vi "Module Loop.vi"(8 "error in (no error)":errorcluster, 11 "Log Manager Module in":refnum<class "Log Manager Module.lvclass">) -> (0 "error out":errorcluster, 3 "Log Manager Module out":refnum<class "Log Manager Module.lvclass">)   [LabVIEW 2023, in "VolatusData.lvlib" / "Log Manager Module.lvclass"]
uses:
  Log Manager Module.lvclass
  Volatus/Module/Module.lvclass
  Log Preparer Module/Log Preparer Module.lvclass
  Log Manager Module.lvclass/Log Manager Module.ctl
  lv-cdm/CDM-Config/ISO8601 Config.ctl
  lv-cdm/CDM-Config/Format.ctl
  lv-cdm/CDM-Config/Precision.ctl
  lv-cdm/CDM-Config/Timezone.ctl
  messages/StartLog/Data.ctl
  lv-vecto/Vecto/proto/TcpPayload/Data.ctl
  Volatus/Module/Module.lvclass/Module.ctl
  Volatus/MessageQ/MessageQ.lvclass/MessageQ.ctl
  Volatus/StringValue/StringValue.lvclass/StringValue.ctl
  Register Logger.ctl
  Volatus/MessageQ/MessageQ.lvclass
  messages/StartLog/Class/Msg.lvclass
  messages/StartLog/Class/Msg.lvclass/Msg.ctl
  Logger Ready.ctl
  messages/StopLog/Class/Msg.lvclass
  messages/StopLog/Class/Msg.lvclass/Msg.ctl
  messages/StopLog/Data.ctl
  Logger Started.ctl
  Logger Stopped.ctl
  Unregister Logger.ctl
  Volatus/Module/Self Q.vi
  Volatus/MessageQ/Send.vi
  lv-cdm/CDM-Config/ISO-8601 Format Strings.vi
  lv-promises/Promises/Promise/Promise.lvclass
  Volatus/StringValue/StringValue.lvclass
  VolatusData.lvlib
  lv-cdm/CDM-Config/CDM-Config.lvlib
  messages/StartLog/StartLog.lvlib
  lv-vecto/Vecto/proto/TcpPayload/TcpPayload.lvlib
  Log Status Value/Log Status Value.lvclass
  messages/StopLog/StopLog.lvlib
  C:/dev/volatus/mts-volatus-super/libs/lv-volatus/Volatus/Module/Module.lvclass
  C:/dev/volatus/mts-volatus-super/libs/lv-volatus/VolatusData/Log Manager Module/Log Manager Module.lvclass
  C:/dev/volatus/mts-volatus-super/libs/lv-volatus/messages/StartLog/Class/Msg.lvclass
  C:/dev/volatus/mts-volatus-super/libs/lv-protoc/LV-Proto/Message/Message.lvclass
  C:/dev/volatus/mts-volatus-super/libs/lv-volatus/messages/StopLog/Class/Msg.lvclass
panel:
  in  "Log Series":string
  in  "Log":bool
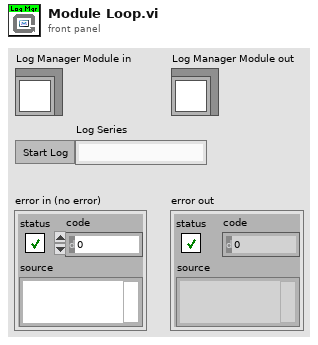
[diagram p1: front panel]
types:
  T1 = enum32{"Invalid", "Standard", "Closed", "Hidden", "Minimized", "Maximized"}
  T2 = typedef "TcpPayload.lvlib/Data.ctl" = cluster{"target_node":u32, "source_id":u32, "sequence":u32, "timestamp":i64, "type":string, "task_id":string, "payload":u8[]}
  T3 = typedef "StartLog.lvlib/Data.ctl" = cluster{"series":string, "timestamp":string, "started_by":string, "groups":string[]}
  T4 = typedef "CDM-Config.lvlib/ISO8601 Config.ctl" = cluster{"Format":T5, "Precision":T6, "Timezone":T7}
  T5 = typedef "CDM-Config.lvlib/Format.ctl" = enum16{"Extended", "Basic"}
  T6 = typedef "CDM-Config.lvlib/Precision.ctl" = enum16{"Millisecond", "Second", "Minute", "Hour", "Day"}
  T7 = typedef "CDM-Config.lvlib/Timezone.ctl" = enum16{"UTC", "Local"}
  T8 = typedef "VolatusData.lvlib/Register Logger.ctl" = cluster{"MsgQ":refnum<class "MessageQ.lvclass">, "ID":string, "Group":string}
  T9 = typedef "VolatusData.lvlib/Logger Ready.ctl" = cluster{"ID":string}
  T10 = typedef "StopLog.lvlib/Data.ctl" = cluster{"reason":string, "groups":string[]}
  T11 = typedef "VolatusData.lvlib/Logger Started.ctl" = cluster{"ID":string}
  T12 = typedef "VolatusData.lvlib/Logger Stopped.ctl" = cluster{"ID":string}
  T13 = typedef "VolatusData.lvlib/Unregister Logger.ctl" = cluster{"ID":string}
  T14 = typedef "VolatusData.lvlib/Log Manager Module.lvclass/Prep Info.ctl" = cluster{"State":T15, "Error":errorcluster}
  T15 = typedef "VolatusData.lvlib/Prep State.ctl" = enum16{"Unknown", "In Progress", "Success", "Failed"}
  T16 = typedef "VolatusData.lvlib/Log Status.ctl" = cluster{"State":T17, "Log":string, "Groups":T18[]}
  T17 = typedef "VolatusData.lvlib/Logging State.ctl" = enum16{"Idle", "Starting", "Logging", "Stopping"}
  T18 = typedef "VolatusData.lvlib/Group State.ctl" = cluster{"Group":string, "State":T19}
  T19 = typedef "VolatusData.lvlib/Logger State.ctl" = enum16{"Unknown", "Idle", "Preparing", "Ready", "Logging", "Stopping"}
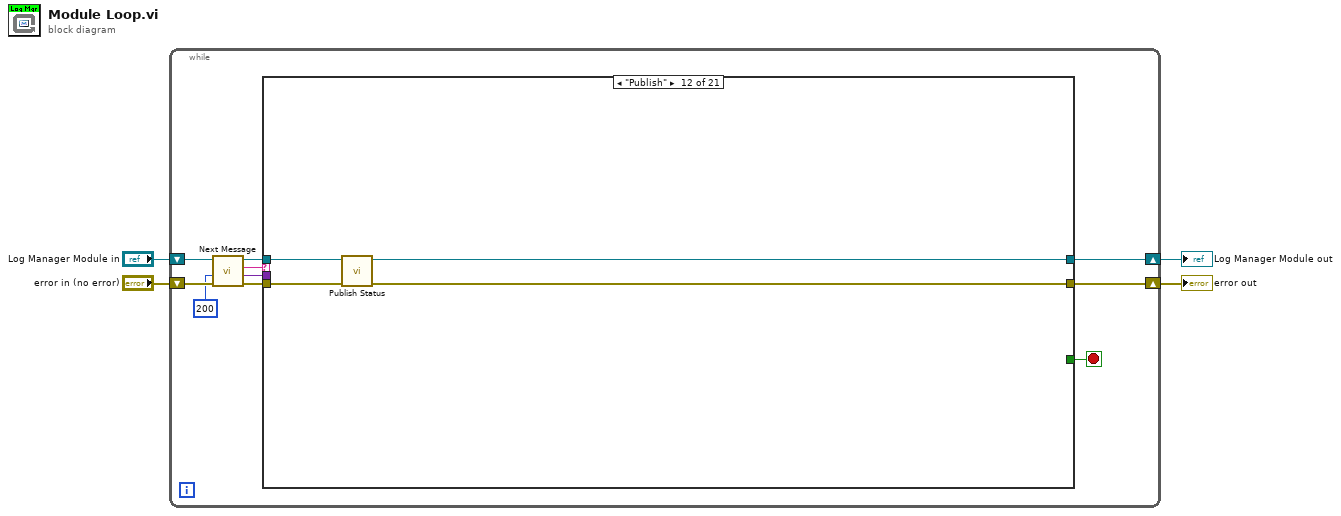
[diagram p0: block diagram]
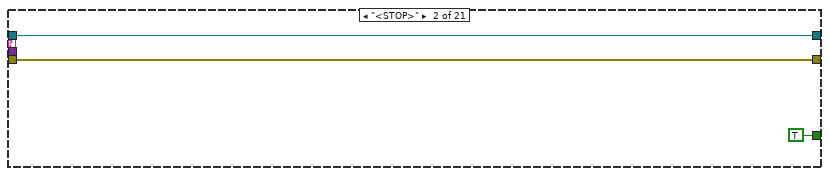
[diagram p3: hidden frame]
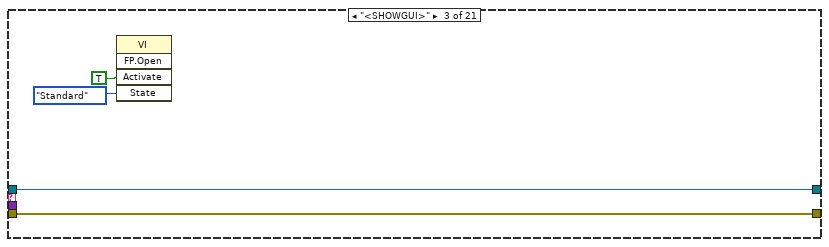
[diagram p4: hidden frame]
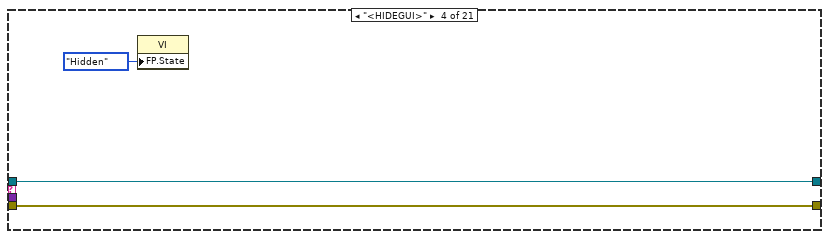
[diagram p5: hidden frame]
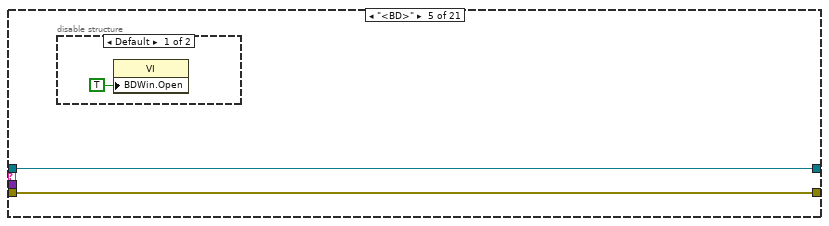
[diagram p6: hidden frame]
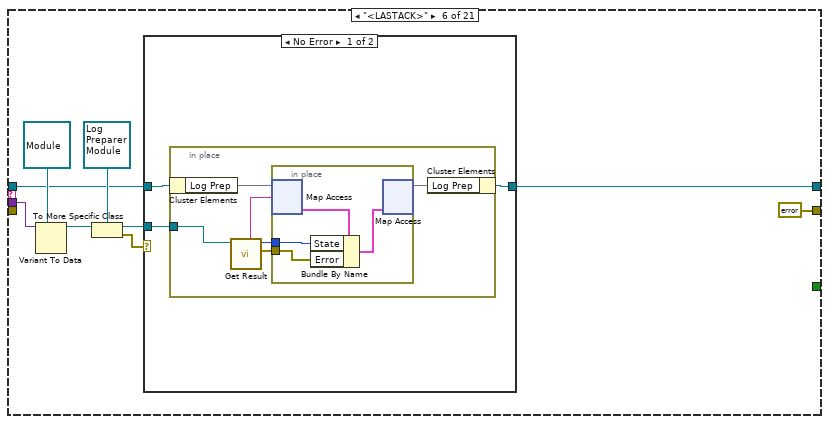
[diagram p8: hidden frame]
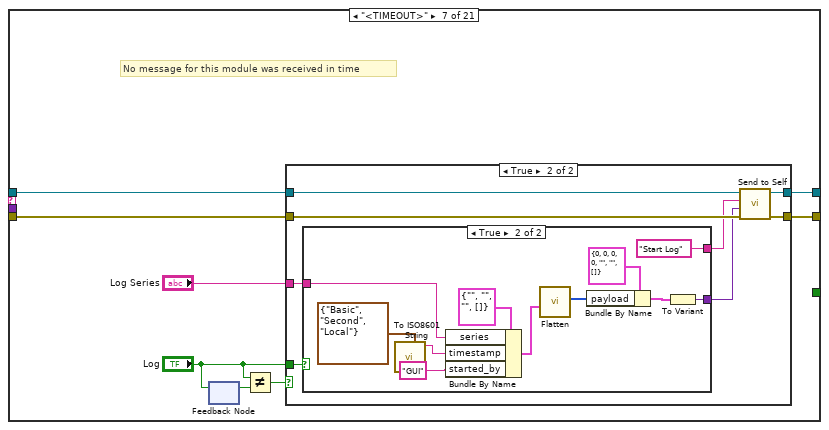
[diagram p10: hidden frame]
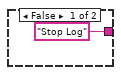
[diagram p12: hidden frame]
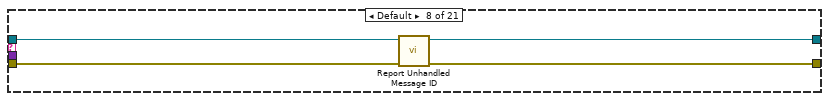
[diagram p13: hidden frame]
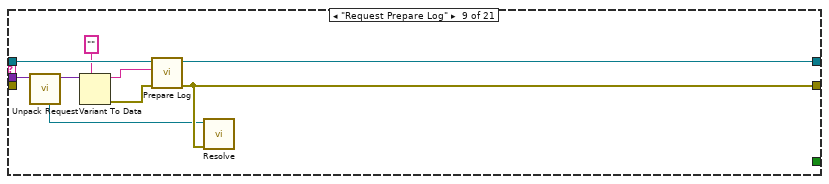
[diagram p14: hidden frame]
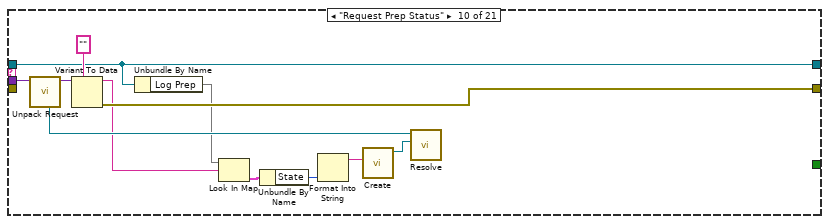
[diagram p15: hidden frame]
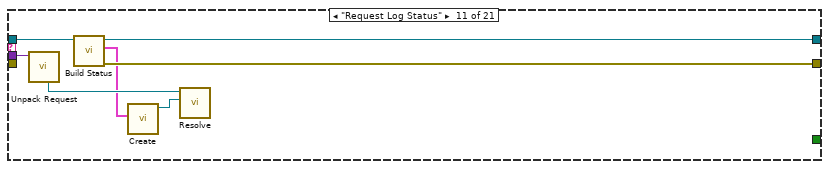
[diagram p16: hidden frame]
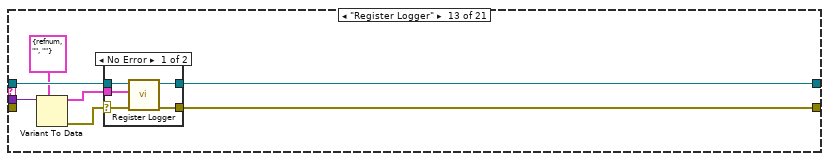
[diagram p17: hidden frame]
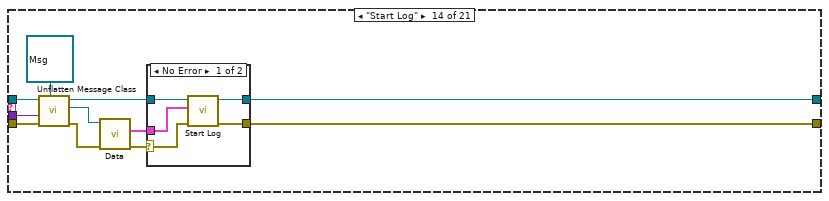
[diagram p19: hidden frame]
diagram:
  n1 = while {
    shift-right: [w9] -> w2
    shift-left: "Log Manager Module in" -> [w14]
    shift-right: [w5] -> w1
    shift-left: "error in (no error)" -> [w13]
    stop <- w8 stop-if-true
    n2 = call "Next Message.vi"("error in (no error)"=w13, "Timeout ms (-1)"=200, "Module in"=w14) -> ("error out"=w12:errorcluster, "Data"=w7:variant, "ID"=w11:string, "Module out"=w10:refnum<class "Log Manager Module.lvclass">)  [unwired: 5 in]
    n3 = case shown="\"Publish\"" w11 {
      tunnel: w12 -> [w15 w18 w22 w25 w27 _ w60 w86 _ _ _ w117 _ w143 _ _ w196 _ _ _ _]
      tunnel: w10 -> [w16 w19 w23 w26 w28 w32 w59 w84 w94 w102 w113 w118 w125 w142 w154 w166 w195 w201 w212 w222 w238]
      tunnel: [w16 w19 w23 w26 w28 w31 w54 w83 w92 w102 w109 w115 w122 w133 w158 w163 w197 w206 w208 w219 w235] -> w9
      tunnel: [_ TRUE _ _ _ _ _ _ _ _ _ _ _ _ _ _ _ _ _ _ _] -> w8
      tunnel: w7 -> [_ _ _ _ _ w38 _ _ w89 w105 w112 _ w124 w141 w157 w165 w188 w205 w215 w221 w237]
      tunnel: [w15 w18 w22 w25 w27 errorcluster {"status"=FALSE, "code"=0, "source"=""} ("error IO") w53 w85 w95 w107 w114 w116 w119 w134 w159 w160 w198 w207 w209 w216 w232] -> w5
      frame "<CLOSE>" {
      }
      frame "<STOP>" {
      }
      frame "<SHOWGUI>" {
        n4 = invoke class="VI" method="FP.Open"("Activate"=TRUE ("Activate?"), "State"=T1."Standard") -> ()  [unwired: 3 in, 5 out]
      }
      frame "<HIDEGUI>" {
        n5 = property class="VI"("FP.State"=T1."Hidden" ("Front Panel Window:State")) -> ()  [unwired: 2 in, 2 out]
      }
      frame "<BD>" {
        n6 = disable-structure shown="Default" {
          frame condition #0 (active) {
            n7 = property class="VI"("BDWin.Open"=TRUE ("Block Diagram Window:Open")) -> ()  [unwired: 2 in, 2 out]
          }
          frame condition #1 {
          }
        }
      }
      frame "<LASTACK>" {
        n8 = Variant To Data(type=refnum<class "Module.lvclass"> refnum ("Volatus:Module"), Variant=w38) -> (data=w36:refnum<class "Module.lvclass">)  [unwired: 1 in, 1 out]
        n9 = To More Specific Class(target class=refnum<class "Log Preparer Module.lvclass"> refnum ("VolatusData:Log Preparer Module.lvclass"), reference=w36) -> (specific class reference=w33:refnum<class "Log Preparer Module.lvclass">, error out=w34:errorcluster)  [unwired: 1 in]
        n10 = case shown="No Error" w34 {
          tunnel: w33 -> [w40 _]
          tunnel: w32 -> [w41 w52]
          tunnel: [w39 w52] -> w31
          frame No Error {
            n11 = in-place {
              in-place-border: w40 -> [w47]
              n12 = in-place-cluster #1(w41) -> ("Log Prep"=w44:map{string, T14})
              n13 = call "Get Result.vi"("Log Preparer Module in"=w47) -> ("error out"=w45:errorcluster, "Result"=w46:T15, "Log"=w43:string)  [unwired: 8 in]
              n14 = in-place {
                in-place-border: w46 -> [w50]
                in-place-border: w45 -> [w51]
                n15 = in-place-map #2(w44, w43) -> (w48:T14)  [unwired: 1 in, 1 out]
                n16 = Bundle By Name(cluster=w48, "State"=w50, "Error"=w51) -> (w49:T14)
                n17 = in-place-map #2(w49) -> (w42:map{string, T14})  [unwired: 1 in, 2 out]
              }
              n18 = in-place-cluster #1("Log Prep"=w42) -> (w39:refnum<class "Log Manager Module.lvclass">)
            }
          }
          frame Error {
          }
        }
      }
      frame "<TIMEOUT>" {
        # "No message for this module was received in time"
        n19 = feedback-in #3("Log") -> ()
        n20 = feedback #3() -> (w58:bool)  [unwired: 1 in]
        n21 = Not Equal?(x="Log", y=w58) -> (x != y?=w57:bool)
        n22 = case shown="True" w57 {
          tunnel: w59 -> [w62 w70]
          tunnel: "Log" -> [_ w63]
          tunnel: "Log Series" -> [_ w66]
          tunnel: w60 -> [w61 w69]
          tunnel: [w62 w68] -> w54
          tunnel: [w61 w67] -> w53
          frame False {
          }
          frame True {
            n23 = case shown="True" w63 {
              tunnel: w66 -> [_ w80]
              tunnel: ["Stop Log" ("Message ID") "Start Log" ("Message ID")] -> w65
              tunnel: [_ w76] -> w64
              frame False {
              }
              frame True {
                n24 = call "To ISO8601 String.vi"("Format Config"=T4 {"Format"=enum."Basic", "Precision"=enum."Second", "Timezone"=enum."Local"}) -> ("ISO 8601"=w79:string)  [unwired: 10 in]
                n25 = Bundle By Name(cluster=T3 {"series"="", "timestamp"="", "started_by"="", "groups"=[]} ("StartLog"), "series"=w80, "timestamp"=w79, "started_by"="GUI") -> (w75:T3)
                n26 = call "Flatten.vi"("Data"=w75) -> ("Buffer"=w72:u8[])  [unwired: 9 in, 1 out]
                n27 = Bundle By Name(cluster=T2 {"target_node"=0, "source_id"=0, "sequence"=0, "timestamp"=0, "type"="", "task_id"="", "payload"=[]} ("TcpPayload"), "payload"=w72) -> (w73:T2)
                n28 = To Variant(anything=w73) -> (Variant=w76:variant)
              }
            }
            n29 = call "Send to Self.vi"("error in (no error)"=w69, "Data"=w64, "Message ID"=w65, "Module in"=w70) -> ("error out"=w67:errorcluster, "Module out"=w68:refnum<class "Log Manager Module.lvclass">)  [unwired: 6 in]
          }
        }
      }
      frame Default {
        n30 = call "Report Unhandled Message ID.vi"("error in (no error)"=w86, "Module in"=w84) -> ("error out"=w85:errorcluster, "Module out"=w83:refnum<class "Log Manager Module.lvclass">)  [unwired: 8 in]
      }
      frame "Request Prepare Log" {
        n31 = call "Unpack Request.vi"("Request Data"=w89) -> ("Data"=w88:variant, "Promise"=w87:refnum<class "Promise.lvclass">)  [unwired: 8 in, 1 out]
        n32 = Variant To Data(type="", Variant=w88) -> (data=w91:string, error out=w90:errorcluster)  [unwired: 1 in]
        n33 = call "Prepare Log.vi"("error in (no error)"=w90, "Log"=w91, "Log Manager Module in"=w94) -> ("error out"=w95:errorcluster, "Log Manager Module out"=w92:refnum<class "Log Manager Module.lvclass">)  [unwired: 7 in]
        n34 = call "Resolve.vi"("error in (no error)"=w95, "Promise in"=w87) -> ()  [unwired: 8 in, 2 out]
      }
      frame "Request Prep Status" {
        n35 = call "Unpack Request.vi"("Request Data"=w105) -> ("Data"=w104:variant, "Promise"=w103:refnum<class "Promise.lvclass">)  [unwired: 8 in, 1 out]
        n36 = Variant To Data(type="", Variant=w104) -> (data=w100:string, error out=w107:errorcluster)  [unwired: 1 in]
        n37 = Unbundle By Name(w102) -> ("Log Prep"=w101:map{string, T14})
        n38 = Look In Map(map=w101, key=w100) -> (value=w99:T14)  [unwired: 1 in, 1 out]
        n39 = Unbundle By Name(w99) -> ("State"=w98:T15)
        n40 = Format Into String(w98) -> (resulting string=w97:string)  [unwired: 3 in, 1 out]
        n41 = call "Create.vi"("Value"=w97) -> ("StringValue out"=w96:refnum<class "StringValue.lvclass">)  [unwired: 10 in]
        n42 = call "Resolve.vi"("Result (None)"=w96, "Promise in"=w103) -> ()  [unwired: 8 in, 2 out]
      }
      frame "Request Log Status" {
        n43 = call "Unpack Request.vi"("Request Data"=w112) -> ("Promise"=w111:refnum<class "Promise.lvclass">)  [unwired: 8 in, 2 out]
        n44 = call "Build Status.vi"("Log Manager Module in"=w113) -> ("error out"=w114:errorcluster, "Logging State"=w108:T16, "Log Manager Module out"=w109:refnum<class "Log Manager Module.lvclass">)  [unwired: 8 in]
        n45 = call "Create.vi"("Log Status"=w108) -> ("Log Status Value out"=w110:refnum<class "Log Status Value.lvclass">)  [unwired: 10 in]
        n46 = call "Resolve.vi"("Result (None)"=w110, "Promise in"=w111) -> ()  [unwired: 8 in, 2 out]
      }
      frame "Publish" {
        n47 = call "Publish Status.vi"("error in (no error)"=w117, "Log Manager Module in"=w118) -> ("error out"=w116:errorcluster, "Log Manager Module out"=w115:refnum<class "Log Manager Module.lvclass">)  [unwired: 8 in]
      }
      frame "Register Logger" {
        n48 = Variant To Data(type=T8 {"MsgQ"=refnum, "ID"="", "Group"=""} ("Logger Registration"), Variant=w124) -> (data=w121:T8, error out=w120:errorcluster)  [unwired: 1 in]
        n49 = case shown="No Error" w120 {
          selector: w120 -> [w127 w131]
          tunnel: w125 -> [w130 w132]
          tunnel: [w129 w132] -> w122
          tunnel: w121 -> [w128 _]
          tunnel: [w126 w131] -> w119
          frame No Error {
            n50 = call "Register Logger.vi"("error in (no error)"=w127, "Logger Registration"=w128, "Log Manager Module in"=w130) -> ("error out"=w126:errorcluster, "Log Manager Module out"=w129:refnum<class "Log Manager Module.lvclass">)  [unwired: 7 in]
          }
          frame Error {
          }
        }
      }
      frame "Start Log" {
        n51 = call "Unflatten Message Class.vi"("Message Type"=refnum<class "Msg.lvclass"> refnum ("StartLog.lvlib:Msg.lvclass"), "error in (no error)"=w143, "Data"=w141, "Module in"=w142) -> ("error out"=w139:errorcluster, "Message"=w138:refnum<class "Msg.lvclass">, "Module out"=w135:refnum<class "Log Manager Module.lvclass">)  [unwired: 4 in, 1 out]
        n52 = call "Data.vi"("error in (no error)"=w139, "PB Msg Template in"=w138) -> ("error out"=w137:errorcluster, "Data"=w136:T3)  [unwired: 7 in, 1 out]
        n53 = case shown="No Error" w137 {
          selector: w137 -> [w146 w149]
          tunnel: w136 -> [w147 _]
          tunnel: w135 -> [w148 w150]
          tunnel: [w145 w149] -> w134
          tunnel: [w144 w150] -> w133
          frame No Error {
            n54 = call "Start Log.vi"("error in (no error)"=w146, "Data"=w147, "Log Manager Module in"=w148) -> ("error out"=w145:errorcluster, "Log Manager Module out"=w144:refnum<class "Log Manager Module.lvclass">)  [unwired: 7 in]
          }
          frame Error {
          }
        }
      }
      frame "Request Start Log" {
        n55 = call "Unpack Request.vi"("Request Data"=w157) -> ("Data"=w156:variant, "Promise"=w151:refnum<class "Promise.lvclass">)  [unwired: 8 in, 1 out]
        n56 = Variant To Data(type=T3 {"series"="", "timestamp"="", "started_by"="", "groups"=[]} ("Data"), Variant=w156) -> (data=w153:T3, error out=w152:errorcluster)  [unwired: 1 in]
        n57 = call "Start Log.vi"("error in (no error)"=w152, "Data"=w153, "Log Manager Module in"=w154) -> ("error out"=w159:errorcluster, "Log Manager Module out"=w158:refnum<class "Log Manager Module.lvclass">)  [unwired: 7 in]
        n58 = call "Resolve.vi"("error in (no error)"=w159, "Promise in"=w151) -> ()  [unwired: 8 in, 2 out]
      }
      frame "Logger Ready" {
        n59 = Variant To Data(type=T9 {"ID"=""} ("Logger Ready"), Variant=w165) -> (data=w161:T9, error out=w162:errorcluster)  [unwired: 1 in]
        n60 = case shown="No Error" w162 {
          selector: w162 -> [w172 w186]
          tunnel: w166 -> [w168 w187]
          tunnel: [w169 w187] -> w163
          tunnel: w161 -> [w171 _]
          tunnel: [w170 w186] -> w160
          frame No Error {
            n61 = Unbundle By Name(w168) -> ("State"=w167:T17)
            n62 = case shown="\"Starting\"" w167 {
              selector: w167 -> [w175 _]
              tunnel: w172 -> [_ w185]
              tunnel: w171 -> [_ w184]
              tunnel: [w173 w182] -> w170
              tunnel: [w178 w180] -> w169
              tunnel: w168 -> [w178 w179]
              frame Default {
                n63 = Format Into String(format string="Must be in Starting state to update logger readiness, instead in \"%s\" state.", w175) -> (resulting string=w174:string)  [unwired: 2 in, 1 out]
                n64 = call <vilib>:"Error Cluster From Error Code.vi"("error message (\"\")"=w174, "error code (0)"=-909) -> ("error out"=w173:errorcluster)  [unwired: 7 in]
              }
              frame "Starting" {
                n65 = call "Logger Ready.vi"("error in (no error)"=w185, "Logger Ready"=w184, "Log Manager Module in"=w179) -> ("error out"=w183:errorcluster, "Log Manager Module out"=w181:refnum<class "Log Manager Module.lvclass">)  [unwired: 7 in]
                n66 = call "Start If All Ready.vi"("error in (no error)"=w183, "Log Manager Module in"=w181) -> ("error out"=w182:errorcluster, "Log Manager Module out"=w180:refnum<class "Log Manager Module.lvclass">)  [unwired: 8 in]
              }
            }
          }
          frame Error {
          }
        }
      }
      frame "Stop Log" {
        n67 = call "Unflatten Message Class.vi"("Message Type"=refnum<class "Msg.lvclass"> refnum ("StopLog.lvlib:Msg.lvclass"), "error in (no error)"=w196, "Data"=w188, "Module in"=w195) -> ("error out"=w191:errorcluster, "Message"=w192:refnum<class "Msg.lvclass">, "Module out"=w194:refnum<class "Log Manager Module.lvclass">)  [unwired: 4 in, 1 out]
        n68 = call "Data.vi"("error in (no error)"=w191, "PB Msg Template in"=w192) -> ("error out"=w189:errorcluster, "Data"=w190:T10)  [unwired: 7 in, 1 out]
        n69 = call "Stop Log.vi"("error in (no error)"=w189, "Data"=w190, "Log Manager Module in"=w194) -> ("error out"=w198:errorcluster, "Log Manager Module out"=w197:refnum<class "Log Manager Module.lvclass">)  [unwired: 7 in]
      }
      frame "Request Stop Log" {
        n70 = call "Unpack Request.vi"("Request Data"=w205) -> ("Data"=w204:variant, "Promise"=w200:refnum<class "Promise.lvclass">)  [unwired: 8 in, 1 out]
        n71 = Variant To Data(type=T10 {"reason"="", "groups"=[]} ("Data"), Variant=w204) -> (data=w202:T10, error out=w199:errorcluster)  [unwired: 1 in]
        n72 = call "Stop Log.vi"("error in (no error)"=w199, "Data"=w202, "Log Manager Module in"=w201) -> ("error out"=w207:errorcluster, "Log Manager Module out"=w206:refnum<class "Log Manager Module.lvclass">)  [unwired: 7 in]
        n73 = call "Resolve.vi"("error in (no error)"=w207, "Promise in"=w200) -> ()  [unwired: 8 in, 2 out]
      }
      frame "Logger Started" {
        n74 = Variant To Data(type=T11 {"ID"=""} ("Logger Started"), Variant=w215) -> (data=w213:T11, error out=w210:errorcluster)  [unwired: 1 in]
        n75 = Unbundle By Name(w213) -> ("ID"=w211:string)
        n76 = call "Logger Started.vi"("error in (no error)"=w210, "ID"=w211, "Log Manager Module in"=w212) -> ("error out"=w209:errorcluster, "Log Manager Module out"=w208:refnum<class "Log Manager Module.lvclass">)  [unwired: 7 in]
      }
      frame "Logger Stopped" {
        n77 = Variant To Data(type=T12 {"ID"=""} ("Logger Stopped"), Variant=w221) -> (data=w217:T12, error out=w218:errorcluster)  [unwired: 1 in]
        n78 = case shown="No Error" w218 {
          selector: w218 -> [w227 w230]
          tunnel: w222 -> [w229 w231]
          tunnel: [w225 w231] -> w219
          tunnel: w217 -> [w226 _]
          tunnel: [w223 w230] -> w216
          frame No Error {
            n79 = call "Logger Stopped.vi"("error in (no error)"=w227, "Logger Stopped"=w226, "Log Manager Module in"=w229) -> ("error out"=w224:errorcluster, "Log Manager Module out"=w228:refnum<class "Log Manager Module.lvclass">)  [unwired: 7 in]
            n80 = call "Check All Stopped.vi"("error in (no error)"=w224, "Log Manager Module in"=w228) -> ("error out"=w223:errorcluster, "Log Manager Module out"=w225:refnum<class "Log Manager Module.lvclass">)  [unwired: 7 in, 1 out]
          }
          frame Error {
          }
        }
      }
      frame "Unregister Logger" {
        n81 = Variant To Data(type=T13 {"ID"=""} ("Unregister Logger"), Variant=w237) -> (data=w233:T13, error out=w234:errorcluster)  [unwired: 1 in]
        n82 = case shown="No Error" w234 {
          selector: w234 -> [w241 w244]
          tunnel: w238 -> [w243 w245]
          tunnel: [w242 w245] -> w235
          tunnel: w233 -> [w240 _]
          tunnel: [w239 w244] -> w232
          frame No Error {
            n83 = call "Unregister Logger.vi"("error in (no error)"=w241, "Unregister Logger"=w240, "Log Manager Module in"=w243) -> ("error out"=w239:errorcluster, "Log Manager Module out"=w242:refnum<class "Log Manager Module.lvclass">)  [unwired: 7 in]
          }
          frame Error {
          }
        }
      }
    }
  }
  "error out" <- w1
  "Log Manager Module out" <- w2
